vi "SpeedValueConversion.vi"(8 "error in (no error)":errorcluster, 11 "Motor Value In":dbl) -> (0 "error out":errorcluster, 3 "New to Old Conversion Value Out":dbl)   [LabVIEW 2014]
panel:
  in  "Old":dbl=12.0
  in  "New":dbl=9.0
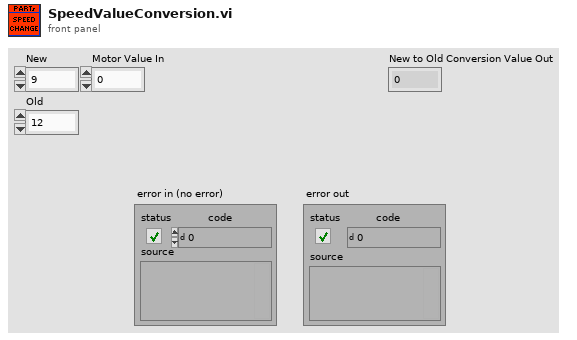
[diagram p1: front panel]
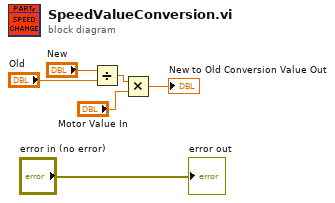
[diagram p0: block diagram]
diagram:
  n1 = Divide(x="New", y="Old") -> (x/y=w4:dbl)
  n2 = Multiply(x=w4, y="Motor Value In") -> (x*y=→"New to Old Conversion Value Out":dbl)
  "error out" <- "error in (no error)"
